vi "PWM Benchmark.vi"() -> ()   [LabVIEW 2013]
uses:
  <vilib>/LabVIEW Hacker/LINX/Private/Type Defs/Peripherals/PWM/PWM Duty Cycle Control.ctl
  <vilib>/LabVIEW Hacker/LINX/Public/Peripherals/PWM/Set Duty Cycle 1 Chan.vi
  <vilib>/ptbypt/NI_PtbyPt.lvlib
  <vilib>/LabVIEW Hacker/LINX/LVH-LINX.lvlib
panel:
  in  "Duty Cycles":T1[](array[typedef])
  in  "Stop Button":bool
  out "Loop Rate":dbl(graph)
  out "Loop Time (ms)":i32
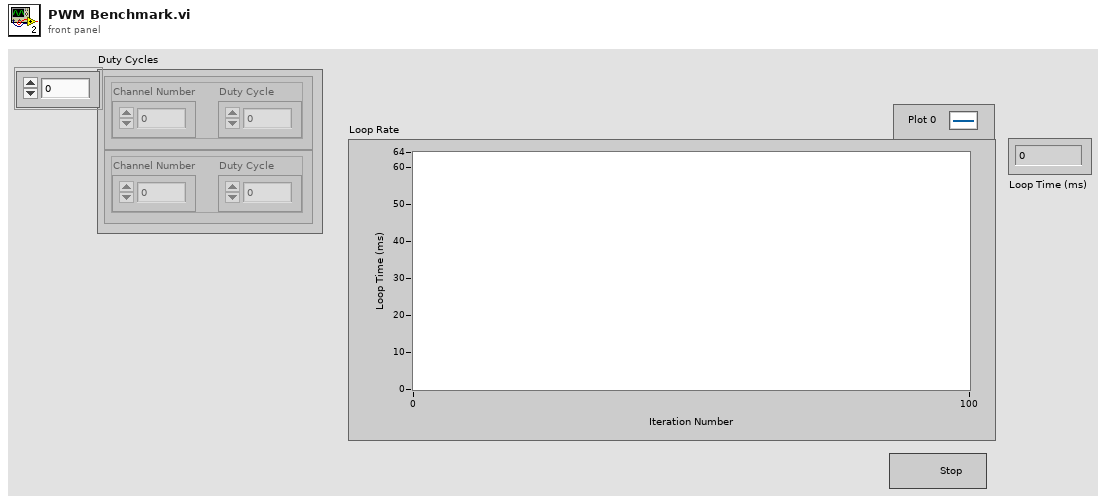
[diagram p1: front panel]
types:
  T1 = typedef "LVH-LINX.lvlib/PWM Duty Cycle Control.ctl" = cluster{"Channel Number":u8, "Duty Cycle":u8}
  T2 = typedef "LVH-LINX.lvlib/LINX Ref.ctl" = cluster{"Platform":T3, "Interface":T4, "LINX Device Config":T5}
  T3 = typedef "LVH-LINX.lvlib/Platform.ctl" = enum16{"LINX", "myRIO"}
  T4 = typedef "LVH-LINX.lvlib/Interface.ctl" = enum16{"Serial", "TCP"}
  T5 = typedef "LVH-LINX.lvlib/Device.lvlib/LINX Device Config.ctl" = cluster{"Interface":T4, "COM Port":refnum<visa-resource-name>, "TCP Configuration":T6, "Device Family":T7, "Device ID":u8, "Device Name":string, "TCP Ref":refnum<k5>}
  T6 = typedef "LVH-LINX.lvlib/Device.lvlib/TCP Config.ctl" = cluster{"IP Address":string, "Port":u16}
  T7 = typedef "LVH-LINX.lvlib/Device Family.ctl" = enum8{"National Instruments", "Digilent", "Arduino"}
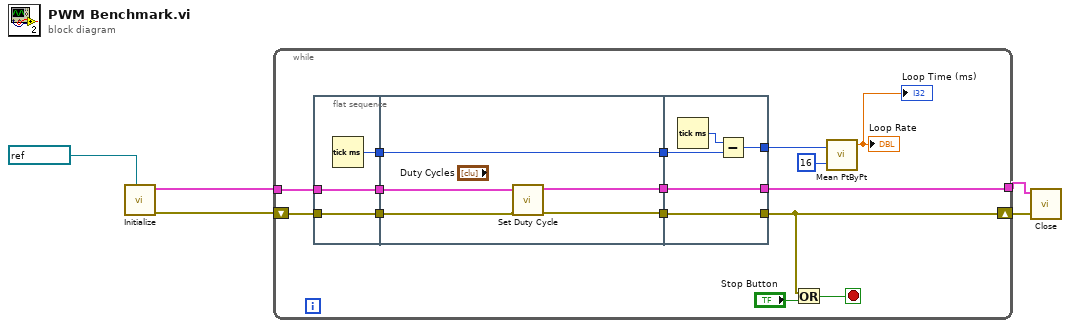
[diagram p0: block diagram]
diagram:
  n1 = call <vilib>:"Initialize.vi"("Serial Port"=refnum<visa-resource-name> "COM5" ("COM Port")) -> ("Error Out"=w1:errorcluster, "LINX Ref"=w5:T2)  [unwired: 8 in, 1 out]
  n2 = while {
    tunnel: w5 -> [w20]
    shift-right: [w6] -> w4
    shift-left: w1 -> [w8]
    tunnel: [w11] -> w3
    stop <- w19 stop-if-true
    n3 = flat-sequence {
      tunnel: w20 -> [w23]
      tunnel: [w23] -> w17
      tunnel: [w22] -> w16
      tunnel: w8 -> [w21]
      tunnel: [w21] -> w7
      tunnel: w17 -> [w24]
      tunnel: w16 -> [w28]
      tunnel: [w28] -> w15
      tunnel: [w27] -> w10
      tunnel: [w26] -> w9
      tunnel: w7 -> [w25]
      tunnel: w15 -> [w32]
      tunnel: [w31] -> w14
      tunnel: [w30] -> w11
      tunnel: w10 -> [w30]
      tunnel: w9 -> [w29]
      tunnel: [w29] -> w6
      frame #0 {
        n4 = Tick Count (ms)() -> (millisecond timer value=w22:u32)
      }
      frame #1 {
        n5 = call-poly <vilib>:"Set Duty Cycle.vi"("Error In"=w25, "LINX Resource"=w24) -> ("Error Out"=w26:errorcluster, "LINX Resource"=w27:T2)  [unwired: 8 in]
      }
      frame #2 {
        n6 = Tick Count (ms)() -> (millisecond timer value=w33:u32)
        n7 = Subtract(x=w33, y=w32) -> (x-y=w31:u32)
      }
    }
    n8 = Or(x=w6, y="Stop Button") -> (x .or. y?=w19:bool)
    n9 = call <vilib>:"Mean PtByPt.vi"("x"=w14, "sample length"=16) -> ("mean"=→"Loop Rate" →"Loop Time (ms)":dbl)  [unwired: 2 in, 1 out]
  }
  n10 = call <vilib>:"Close.vi"("Error In"=w4, "LINX Resource"=w3) -> ()  [unwired: 8 in, 2 out]
